vi "Handle.vi"(7 "Actor in":refnum<class "Actor.lvclass">, 11 "Nominal State in":refnum<class "Nominal State.lvclass">) -> (2 "Destroy?":bool, 5 "Actor out":refnum<class "Actor.lvclass">)   [LabVIEW 2021, in "jettl Event Actor.lvlib" / "Nominal State.lvclass"]
uses:
  Nominal State.lvclass
  Nominal State.lvclass/Nominal State.ctl
  Actor/Actor/Actor.lvclass
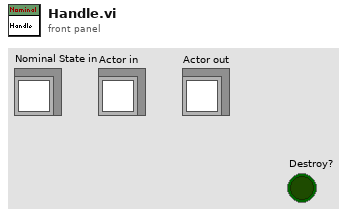
[diagram p1: front panel]
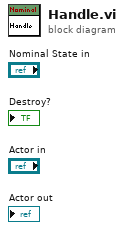
[diagram p0: block diagram]
diagram:
